vi "Destroy CORE UI Display Events.vi"(0 "UI display events in":T1, 11 "error in":errorcluster) -> (15 "error out":errorcluster)   [LabVIEW 2015, in "TLB` Template.lvlib"]
doc: "Close user event resources.\n\n<B>Input Parameters</B>\n\n<B>UI display events in</B> references.\n\n<B>error in</B> describes error conditions that occur before this node runs. This input provides standard error in functionality.\n\n<B>Output Parameters</B>\n\n<B>error out</B> contains error information. This output provides standard error out functionality."
uses:
  TLB` Template.lvlib
  typedefs/_UI CORE Event References.ctl
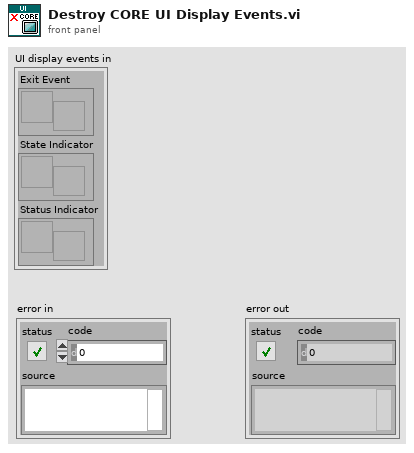
[diagram p1: front panel]
types:
  T1 = typedef "TLB` Template.lvlib/_UI CORE Event References.ctl" = cluster{"Exit Event":refnum<user-event>, "State Indicator":refnum<user-event>, "Status Indicator":refnum<user-event>}
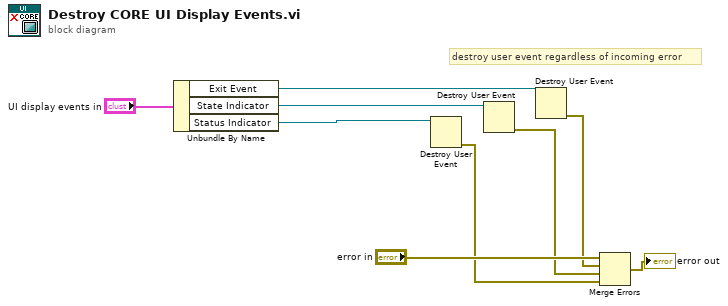
[diagram p0: block diagram]
diagram:
  # "destroy user event regardless of incoming error"
  n1 = Unbundle By Name("UI display events in") -> ("Exit Event"=w4:refnum<user-event>, "State Indicator"=w8:refnum<user-event>, "Status Indicator"=w5:refnum<user-event>)
  n2 = Destroy User Event(user event=w5) -> (error out=w1:errorcluster)  [unwired: 1 in]
  n3 = Destroy User Event(user event=w8) -> (error out=w2:errorcluster)  [unwired: 1 in]
  n4 = Destroy User Event(user event=w4) -> (error out=w3:errorcluster)  [unwired: 1 in]
  n5 = Merge Errors("error in", w3, w2, w1) -> (→"error out":errorcluster)
